vi "MotorOutputs.vi"(7 "Max Wheel Speed":dbl, 8 "error in (no error)":errorcluster, 9 "Motor Speeds":dbl[](array[numeric]), 10 "Target Angles":dbl[](array[numeric]), 11 "Steering Refnums In":T10) -> (0 "error out":errorcluster, 1 "Speed Motor Setpoints":dbl[](array[numeric]), 2 "Steering Motor Setpoints":dbl[](array[numeric]), 3 "Steering Refnums Out":T10)   [LabVIEW 2014]
uses:
  <vilib>/Rock Robotics/WPI/MotorControl/WPI_MotorControlDeviceRef.ctl
  <vilib>/Rock Robotics/WPI/MotorControl/WPI_MotorControlType.ctl
  <vilib>/Rock Robotics/SystemInterfaces/Typedef/FPGA_TypedefDigitalModule.ctl
  <vilib>/Rock Robotics/SystemInterfaces/DIO/FPGA_DIOPWMChannel.ctl
  <vilib>/Rock Robotics/WPI/PWM/WPI_PWMDeadband.ctl
  <vilib>/Rock Robotics/WPI/CAN/Jaguar/SubVIs/WPI_CANJaguar_ControlMode.ctl
  <vilib>/Rock Robotics/WPI/CAN/TalonSRX/WPI_CANTalonSRX_APIControlMode.ctl
  <vilib>/Rock Robotics/WPI/PWM/WPI_PWMTransform_ConPane.ctl
  Robot Global Data.vi
panel:
  out "Speed Cluster":T11 {"RR Speed" scale=-1.0..1.0; "RL Speed" scale=-1.0..1.0; "FR Speed" scale=-1.0..1.0; "FL Speed" scale=-1.0..1.0}
  out "Angle Cluster":T12 {"FL Angle" scale=3.1416..-3.1416; "FR Angle" scale=3.1416..-3.1416; "RR Angle" scale=3.1416..-3.1416; "RL Angle" scale=3.1416..-3.1416}
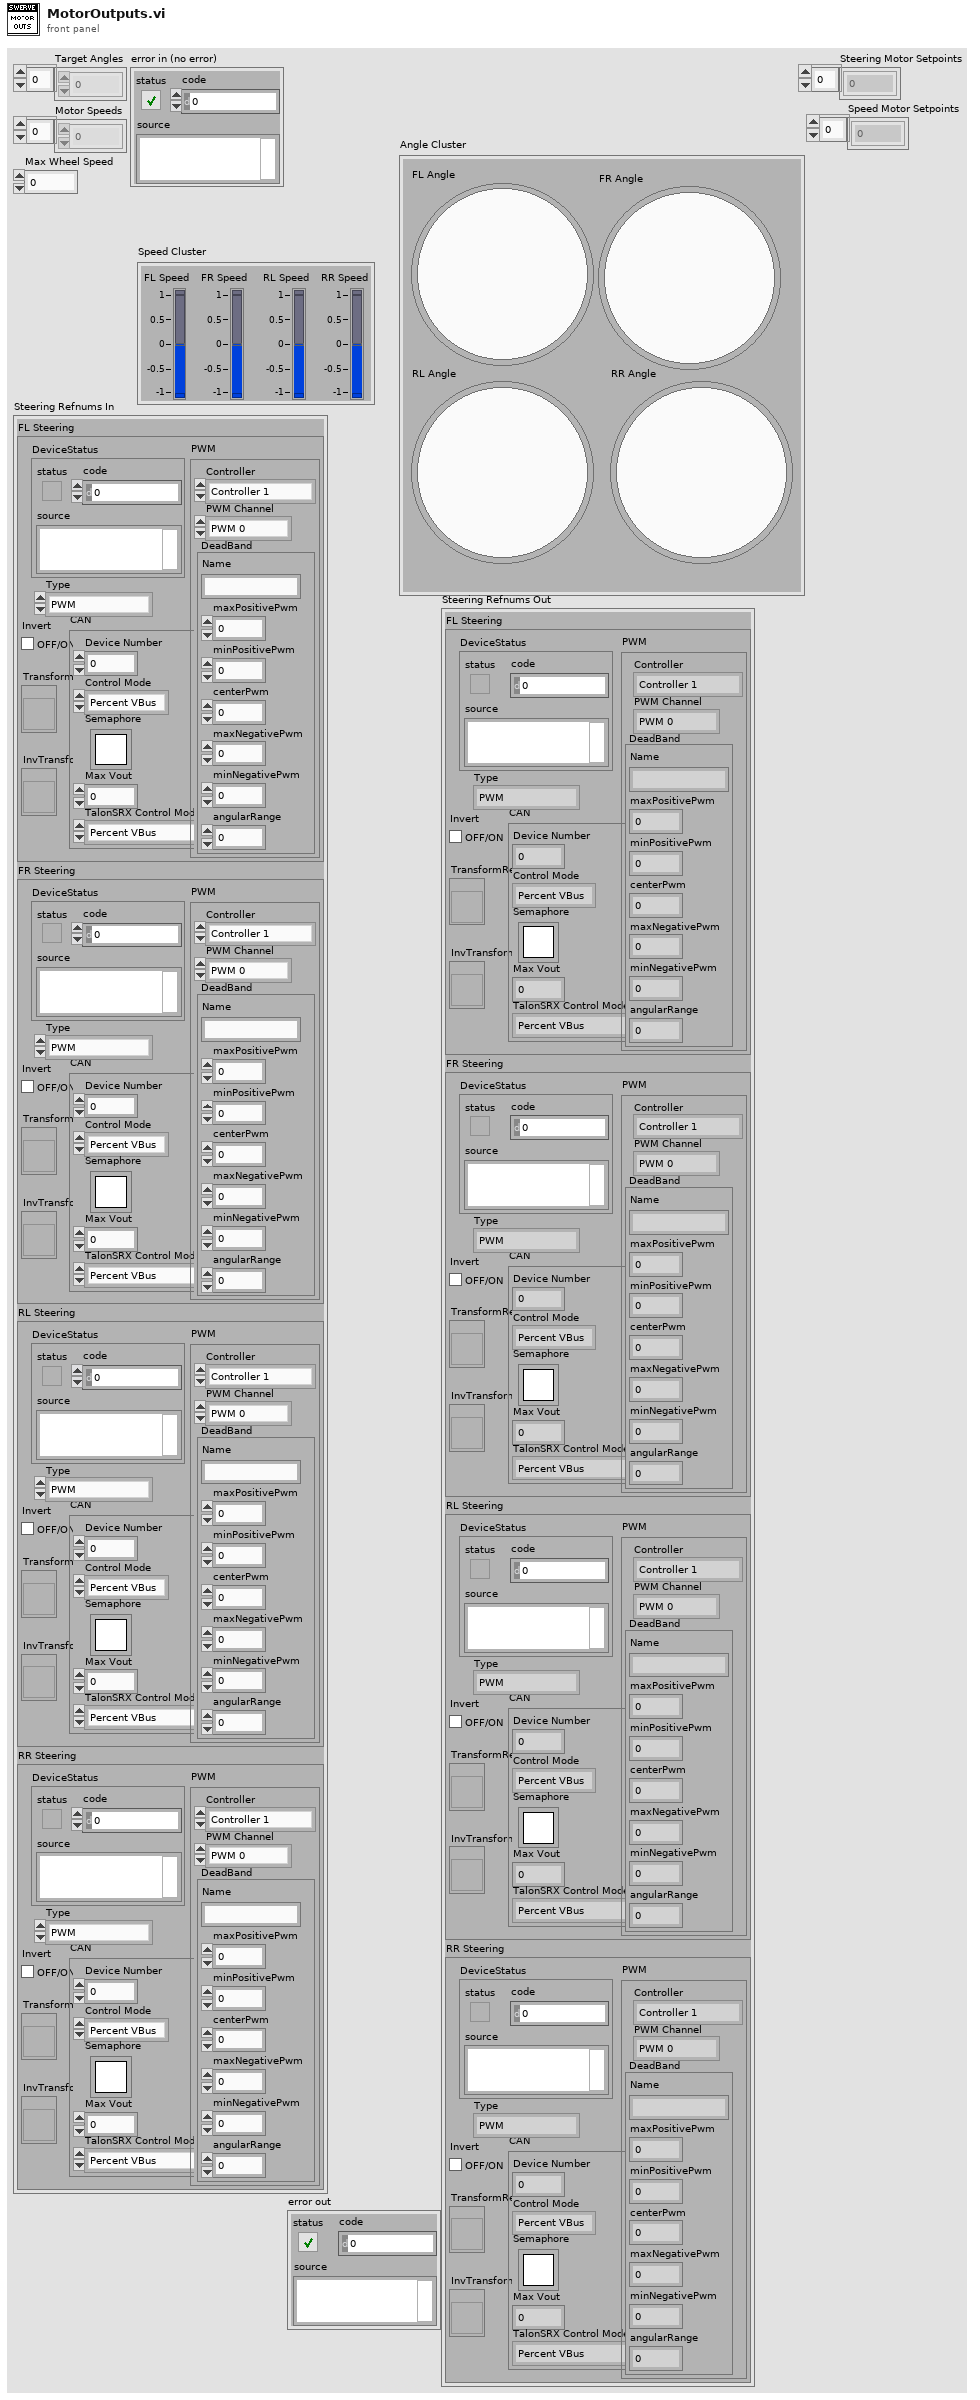
[diagram p1: front panel]
types:
  T1 = typedef "WPI_MotorControlDeviceRef.ctl" = cluster{"DeviceStatus":errorcluster, "Type":T2, "PWM":cluster{"Controller":T3, "PWM Channel":T4, "DeadBand":T5}, "CAN":cluster{"Device Number":u8, "Control Mode":T6, "Semaphore":T7, "Max Vout":dbl, "TalonSRX Control Mode":T8}, "Invert":bool, "TransformRef":T9, "InvTransformRef":T9}
  T2 = typedef "WPI_MotorControlType.ctl" = enum16{"PWM", "CAN", "CANTalonSRX"}
  T3 = typedef "FPGA_TypedefDigitalModule.ctl" = enum16{"Controller 1"}
  T4 = typedef "FPGA_DIOPWMChannel.ctl" = enum8{"PWM 0", "PWM 1", "PWM 2", "PWM 3", "PWM 4", "PWM 5", "PWM 6", "PWM 7", "PWM 8", "PWM 9", "PWM MXP 0", "PWM MXP 1", "PWM MXP 2", "PWM MXP 3", "PWM MXP 4", "PWM MXP 5", "PWM MXP 6", "PWM MXP 7", "PWM MXP 8", "PWM MXP 9", "Invalid"}
  T5 = typedef "WPI_PWMDeadband.ctl" = cluster{"Name":string, "maxPositivePwm":i32, "minPositivePwm":i32, "centerPwm":i32, "maxNegativePwm":i32, "minNegativePwm":i32, "angularRange":u16}
  T6 = typedef "WPI_CANJaguar_ControlMode.ctl" = enum8{"Percent VBus", "Current", "Speed", "Position", "Voltage"}
  T7 = typedef "Semaphore RefNum" = refnum<k1>
  T8 = typedef "WPI_CANTalonSRX_APIControlMode.ctl" = enum8{"Percent VBus", "Speed", "Position", "Slave", "Unchanged / Invalid"}
  T9 = typedef "WPI_PWMTransform_ConPane.ctl" = refnum<vi>
  T10 = cluster{"FL Steering":T1, "FR Steering":T1, "RL Steering":T1, "RR Steering":T1}
  T11 = cluster{"FL Speed":dbl, "FR Speed":dbl, "RL Speed":dbl, "RR Speed":dbl}
  T12 = cluster{"FL Angle":dbl, "FR Angle":dbl, "RL Angle":dbl, "RR Angle":dbl}
  T13 = cluster{"[0]":dbl, "[1]":dbl, "[2]":dbl, "[3]":dbl}
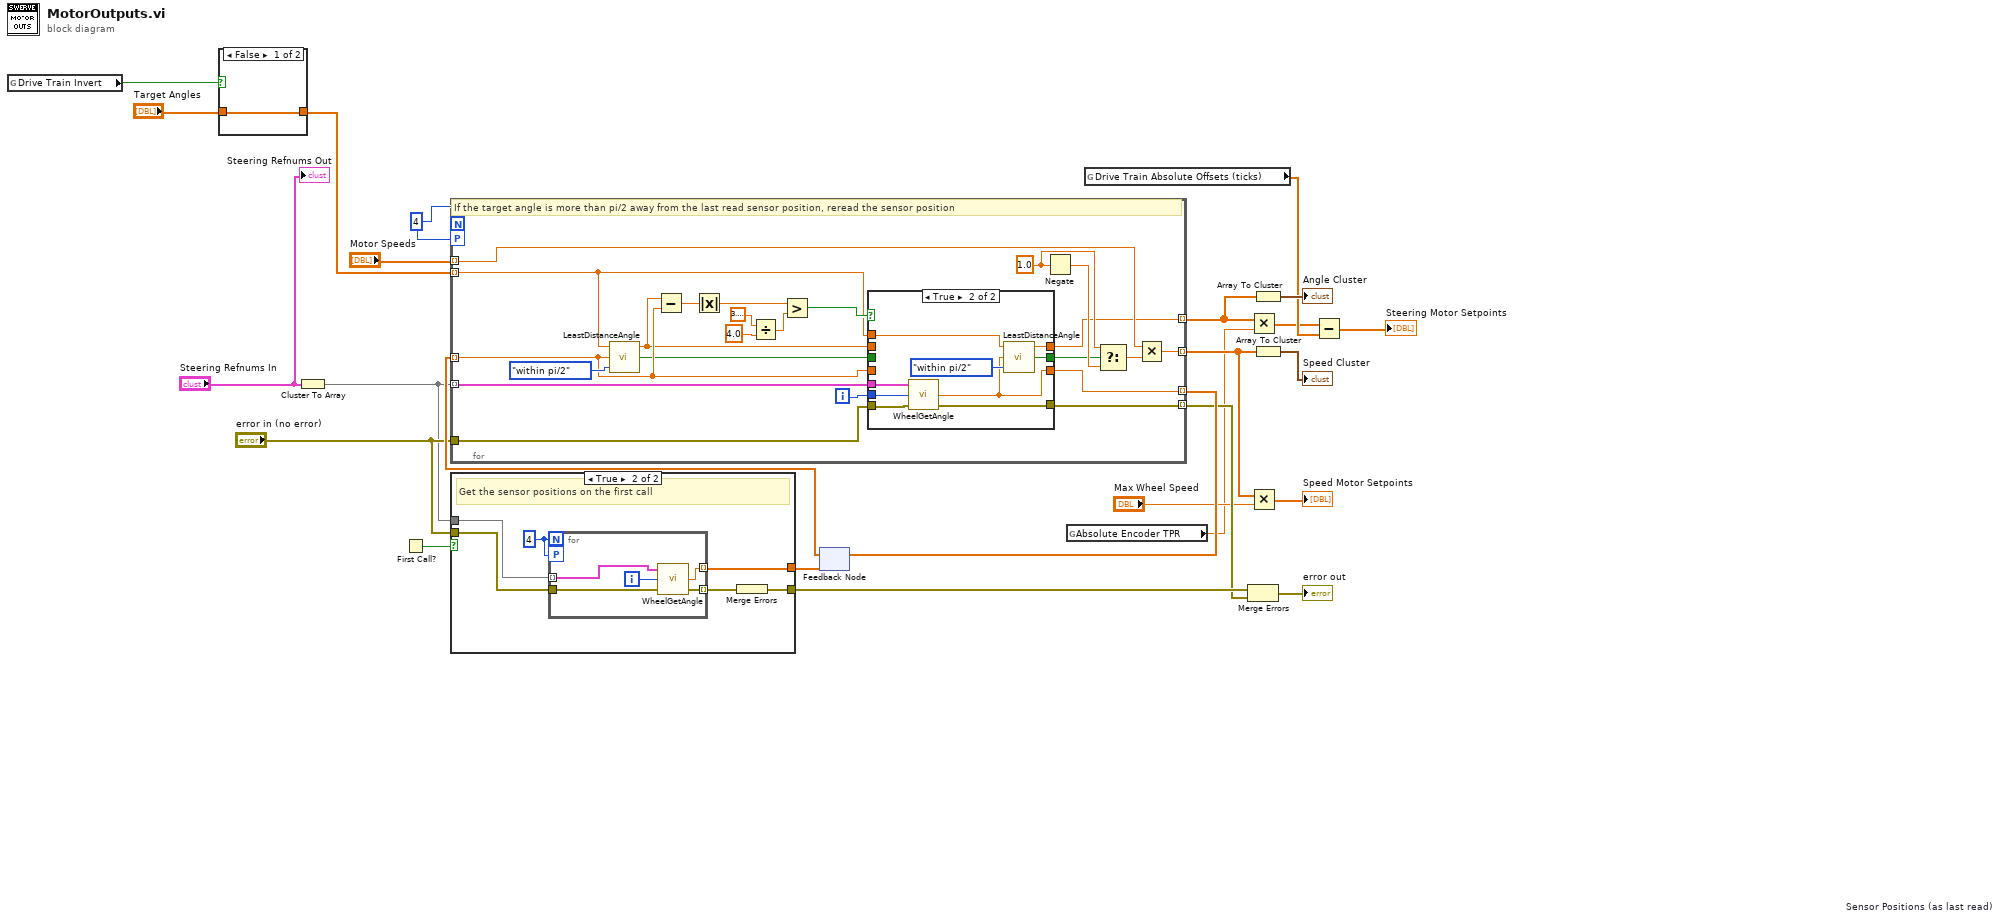
[diagram p0: block diagram]
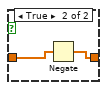
[diagram p2: hidden frame]
diagram:
  w25 = 4
  n1 = global read "Robot Global Data.vi" "Drive Train Invert"() -> (w1:bool)
  n2 = case shown="False" w1 {
    tunnel: "Target Angles" -> [w26 w28]
    tunnel: [w26 w27] -> w2
    frame False {
    }
    frame True {
      n3 = Negate(x=w28) -> (-x=w27:dbl[])
    }
  }
  n4 = Cluster To Array(cluster="Steering Refnums In") -> (array=w16:T1[])
  n5 = First Call?() -> (First Call?: T/F=w22:bool)
  n6 = case shown="True" w22 {
    tunnel: "error in (no error)" -> [w29 w35]
    tunnel: [w29 w34] -> w21
    tunnel: w16 -> [_ w33]
    tunnel: [_ w32] -> w15
    frame False {
    }
    frame True {
      w30 = 4
      # "Get the sensor positions on the first call"
      n7 = for {
        N: w30 -> [_]
        tunnel: [w39] -> w32 mode=indexing
        tunnel: w35 -> [w40]
        tunnel: [w38] -> w31 mode=indexing
        workers-P: w30 -> [_]
        tunnel: w33 -> [w37] mode=indexing
        i -> [w36]
        n8 = call "WheelGetAngle.vi"("error in (no error)"=w40, "Wheel"=w36, "CAN Talon SRX Ref"=w37) -> ("error out"=w38:errorcluster, "Sensor Position (rad)"=w39:dbl)  [unwired: 1 out]
      }
      n9 = Merge Errors(w31) -> (w34:errorcluster)
    }
  }
  n10 = feedback #1 "Sensor Positions (as last read)"(w15) -> (w23:dbl[])
  n11 = for {
    N: w25 -> [_]
    workers-P: w25 -> [_]
    tunnel: [w63] -> w24 mode=indexing
    tunnel: w2 -> [w41] mode=indexing
    tunnel: w23 -> [w52] mode=indexing
    tunnel: "error in (no error)" -> [w62]
    tunnel: [w61] -> w18 mode=indexing
    tunnel: w16 -> [w59] mode=indexing
    tunnel: "Motor Speeds" -> [w47] mode=indexing
    tunnel: [w46] -> w9 mode=indexing
    tunnel: [w44] -> w5 mode=indexing
    i -> [w58]
    w50 = 1.0 ("t")
    # "If the target angle is more than pi/2 away from the last read sensor position, reread the sensor position"
    n12 = call "LeastDistanceAngle.vi"("Enum"=enum16{"within pi", "within pi/2"}."within pi/2", "Current angle"=w52, "target angle (between pi and -pi) 2"=w41) -> ("Reverse?"=w42:bool, "output angle"=w45:dbl)  [unwired: 1 out]
    n13 = Subtract(x=w45, y=w52) -> (x-y=w51:dbl)
    n14 = Absolute Value(x=w51) -> (abs(x)=w57:dbl)
    n15 = Divide(x=3.141592653589793, y=4.0) -> (x/y=w54:dbl)
    n16 = Greater?(x=w57, y=w54) -> (0:w60:bool)
    n17 = case shown="True" w60 {
      tunnel: [w67 w71] -> w63
      tunnel: w52 -> [w67 _]
      tunnel: w62 -> [w66 w74]
      tunnel: [w66 w73] -> w61
      tunnel: w59 -> [_ w76]
      tunnel: w58 -> [_ w75]
      tunnel: w45 -> [w65 _]
      tunnel: [w65 w68] -> w44
      tunnel: [w64 w69] -> w43
      tunnel: w42 -> [w64 _]
      tunnel: w41 -> [_ w70]
      frame False {
      }
      frame True {
        n18 = call "WheelGetAngle.vi"("error in (no error)"=w74, "Wheel"=w75, "CAN Talon SRX Ref"=w76) -> ("error out"=w73:errorcluster, "Sensor Position (rad)"=w71:dbl)  [unwired: 1 out]
        n19 = call "LeastDistanceAngle.vi"("Enum"=enum16{"within pi", "within pi/2"}."within pi/2", "Current angle"=w71, "target angle (between pi and -pi) 2"=w70) -> ("Reverse?"=w69:bool, "output angle"=w68:dbl)  [unwired: 1 out]
      }
    }
    n20 = Negate(x=w50) -> (-x=w49:dbl)
    n21 = Select(t=w50, s=w43, f=w49) -> (s? t:f=w48:dbl)
    n22 = Multiply(x=w47, y=w48) -> (x*y=w46:dbl)
  }
  n23 = feedback-in #1(w24) -> ()
  n24 = global read "Robot Global Data.vi" "Absolute Encoder TPR"() -> (w7:dbl)
  n25 = global read "Robot Global Data.vi" "Drive Train Absolute Offsets (ticks)"() -> (w4:dbl[])
  n26 = Merge Errors(w21, w18) -> (→"error out":errorcluster)
  n27 = Multiply(x=w5, y=w7) -> (x*y=w3:dbl[])
  n28 = Multiply(x=w9, y="Max Wheel Speed") -> (x*y=→"Speed Motor Setpoints":dbl[])
  n29 = Array To Cluster(array=w5) -> (cluster=→"Angle Cluster":T13)
  n30 = Array To Cluster(array=w9) -> (cluster=→"Speed Cluster":T13)
  n31 = Subtract(x=w3, y=w4) -> (x-y=→"Steering Motor Setpoints":dbl[])
  "Steering Refnums Out" <- "Steering Refnums In"
